vi "Fetch Waveform.vi"(0 "CS++Scope":refnum<class "CS++Scope.lvclass">, 1 "channel name (\"CHANNEL1\")":string="CHANNEL1", 2 "waveform size (0)":i32=1000, 5 "error in (no error)":errorcluster) -> (14 "CS++Scope out":refnum<class "CS++Scope.lvclass">, 15 "actual points":i32, 16 "initial x":dbl[unit] format="%^.2e", 17 "x increment":dbl[unit] format="%^.2e", 18 "WaveformArray":waveform(dbl), 19 "error out":errorcluster)   [LabVIEW 2014, in "CS++Scope.lvlib" / "CS++Scope.lvclass"]
doc: "This VI returns the waveform the oscilloscope acquires for the channel you specify. The waveform is from an acquisition that you initiate prior to calling this VI.\n\nThe VI also publishes a variable called MeasurementDone once all channels were updated since the last Init. Nevertheless one should still compare the time stamps of the acquired waveforms.\n\nYou use the IviScope Initiate Acquisition VI to start an acquisition on the channels that you enable with the IviScope Configure Channel VI. The oscilloscope acquires waveforms for the enabled channels concurrently. You use the IviScope Acquisition Status VI to determine when the acquisition is complete. You must call this VI separately for each enabled channel to obtain the waveforms.\n\nYou can call the IviScope Read Waveform VI instead of the IviScope Initiate Acquisition VI. The IviScope Read Waveform VI starts an acquisition on all enabled channels, waits for the acquisition to complete, and returns the waveform for the channel you specify. You call this VI to obtain the waveforms for each of the remaining channels.\n\nNotes:\n\n(1) After this VI executes, each element in the Waveform Array parameter is either a voltage or a value indicating that the oscilloscope could not sample a voltage.\n\n(2) You configure the interpolation method the oscilloscope uses with the IviScope Configure Interpolation [I] VI. If you disable interpolation, the oscilloscope does not interpolate points in the waveform. If the oscilloscope cannot sample a value for a point in the waveform, the driver sets the corresponding element in the Waveform Array to an IEEE defined NaN (Not a Number) value and the VI returns IVISCOPE_WARN_INVALID_WFM_ELEMENT (0x3FFA2001). \n\n(3) You can test a waveform value for an invalid value condition by calling the IviScope Is Invalid Waveform Element VI.\n\n(4) This VI does not check the instrument status. Typically, you call this VI only in a sequence of calls to other low-level driver VIs. The sequence performs one operation. You use the low-level VIs to optimize one or more aspects of interaction with the instrument. If you want to check the instrument status, call the IviScope Error-Query VI at the conclusion of the sequence.\n\n(5) The class driver returns a simulated waveform when this\nVI is called and the IviScope>>Inherent IVI Settings>>User Options>>Simulate property is set to TRUE and the IviScope>>Inherent IVI Settings>>User Options>>Use Specific Simulation property is set to FALSE. For information on how to configure a simulated waveform, refer to the online help manual."
uses:
  CS++Scope.lvclass
  CS++Scope.lvclass/CS++Scope.ctl
  CSPP_Core/Classes/CS++ProcessVariables/ProcessVariable/PV.lvclass
  PV-Enum.ctl
  CSPP_Core/Classes/CS++ProcessVariables/ProcessVariable/PV.lvclass/PV.ctl
  CSPP_Core/Classes/CS++ProcessVariables/ProcessVariable/Write Data.vi
  CSPP_Core/Classes/CS++ProcessVariables/ProcessVariable/Write Timestamp.vi
  CSPP_Core/Classes/CS++ProcessVariables/ProcessVariable/Write Quality.vi
  CSPP_Core/Classes/CS++ProcessVariables/ProcessVariable/Write status.vi
  CSPP_Core/Classes/CS++ProcessVariables/PVConnection/PVConnection.lvclass
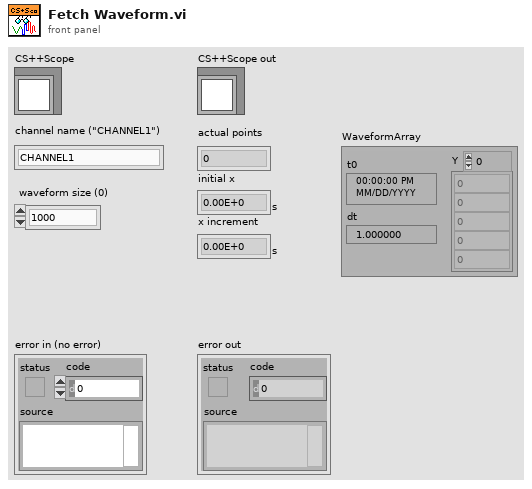
[diagram p1: front panel]
types:
  T1 = typedef "CS++Scope.lvlib/CS++Scope.lvclass/PV-Enum.ctl" = enum16{"ActualSampleRate", "TimePerRecord", "AcquisitionStartTime", "TriggerLevel", "GlitchWidth", "LowReference", "MidReference", "HighReference", "RuntLowThreshold", "RuntHighThreshold", "TriggerHoldoff", "WidthLowThreshold", "WidthHighThreshold", "AcquisitionStatus", "ActualRecordLength", "ActualSampleMode", "ACLineTriggerSlope", "MinRecordLength", "AcquisitionType", "TriggerSlope", "GlitchCondition", "GlitchPolarity", "InterpolationMethod", "NumberOfAverages", "NumberOfEnvelopes", "TriggerType", "TriggerCoupling", "TriggerModifier", "TVLineNumber", "TVEvent", "TVTriggerPolarity", "TVSignalFormat", "WidthCondition", "WidthPolarity", "MeasurementDone", "ContinousAcquisition", "TriggerSource", "Waveform", "ActualTimeIncrement"}
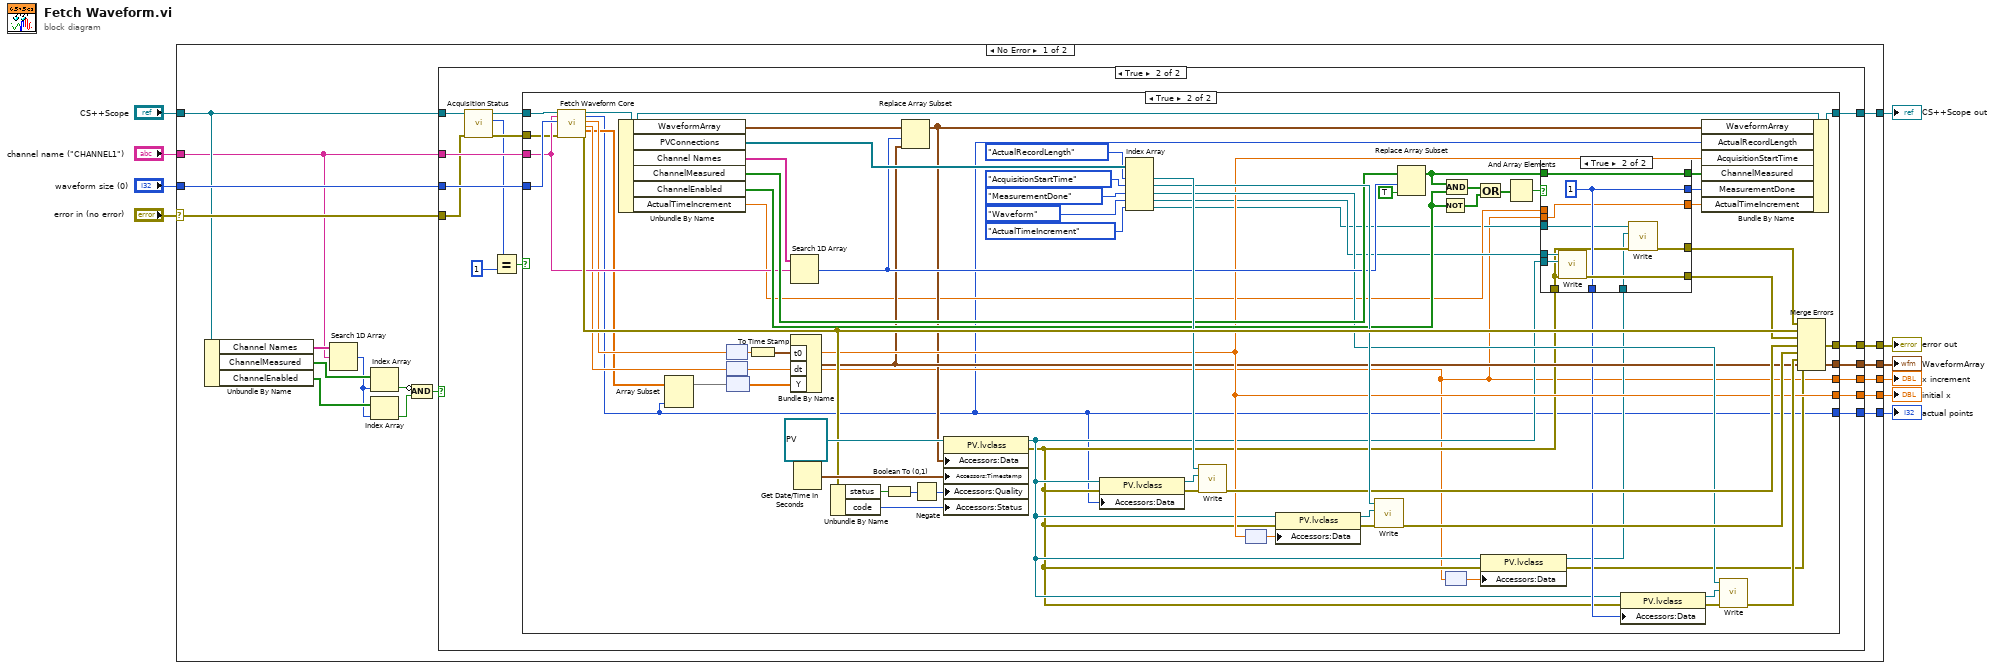
[diagram p0: block diagram]
diagram:
  n1 = case shown="No Error" "error in (no error)" {
    selector: "error in (no error)" -> [w27 w130]
    tunnel: [w26 w130] -> w9
    tunnel: [w22 w129] -> w6
    tunnel: "CS++Scope" -> [w19 w129]
    tunnel: "channel name (\"CHANNEL1\")" -> [w17 _]
    tunnel: "waveform size (0)" -> [w23 _]
    tunnel: [w21 _] -> w1
    tunnel: [w25 _] -> w4
    tunnel: [w20 _] -> w3
    tunnel: [w24 _] -> w2
    frame No Error {
      n2 = Unbundle By Name(w19) -> ("Channel Names"=w18:string[], "ChannelMeasured"=w16:bool[], "ChannelEnabled"=w15:bool[])
      n3 = Search 1D Array(1D array=w18, element=w17) -> (index of element=w14:i32)  [unwired: 1 in]
      n4 = Index Array(array=w16, index=w14) -> (element=w13:bool)
      n5 = Index Array(array=w15, index=w14) -> (element=w12:bool)
      n6 = Compound Arithmetic op=AND(invert w13, w12) -> (w11:bool)
      n7 = case shown="True" w11 {
        tunnel: w27 -> [w28 w34]
        tunnel: [w28 w44] -> w26
        tunnel: [_ w43] -> w25
        tunnel: [_ w42] -> w24
        tunnel: w23 -> [_ w41]
        tunnel: [w29 w40] -> w22
        tunnel: [_ w39] -> w21
        tunnel: [_ w38] -> w20
        tunnel: w19 -> [w29 w36]
        tunnel: w17 -> [_ w37]
        frame False {
        }
        frame True {
          n8 = call "Acquisition Status.vi"("error in (no error)"=w34, "CS++Scope"=w36) -> ("error out"=w33:errorcluster, "acquisition status"=w32:i32, "CS++Scope out"=w35:refnum<class "CS++Scope.lvclass">)  [unwired: 7 in]
          n9 = Equal?(x=w32, y=1) -> (x = y?=w30:bool)
          n10 = case shown="True" w30 {
            tunnel: [w46 w96] -> w44
            tunnel: [_ w47] -> w43
            tunnel: [_ w50] -> w42
            tunnel: w41 -> [_ w95]
            tunnel: [w45 w85] -> w40
            tunnel: [_ w68] -> w39
            tunnel: [_ w71] -> w38
            tunnel: w37 -> [_ w75]
            tunnel: w35 -> [w45 w74]
            tunnel: w33 -> [w46 w73]
            frame False {
            }
            frame True {
              n11 = call-dynamic "Fetch Waveform Core.vi"("CS++Scope"=w74, "channel name (\"CHANNEL1\")"=w75, "waveform size (0)"=w95, "error in (no error)"=w73) -> ("CS++Scope out"=w86:refnum<class "CS++Scope.lvclass">, "actual points"=w47:i32, "initial x"=w71:dbl[unit], "x increment"=w50:dbl[unit], "waveform array"=w49:dbl[unit][], "error out"=w107:errorcluster)  [unwired: 10 in]
              n12 = Unbundle By Name(w86) -> ("WaveformArray"=w114:waveform(dbl)[], "PVConnections"=w104:refnum<class "PVConnection.lvclass">[], "Channel Names"=w115:string[], "ChannelMeasured"=w94:bool[], "ChannelEnabled"=w91:bool[], "ActualTimeIncrement"=w60:dbl[unit])
              n13 = Array Subset(array=w49, length=w47) -> (w48:dbl[unit][])  [unwired: 1 in]
              n14 = node(w71) -> (w70:dbl)
              n15 = node(w50) -> (w59:dbl)
              n16 = node(w48) -> (w69:dbl[])
              n17 = To Time Stamp(1:w70) -> (0:w72:timestamp)
              n18 = Search 1D Array(1D array=w115, element=w75) -> (index of element=w93:i32)  [unwired: 1 in]
              n19 = Bundle By Name("t0"=w72, "dt"=w59, "Y"=w69) -> (w68:waveform(dbl))  [unwired: 1 in]
              n20 = Get Date/Time In Seconds() -> (seconds since 1Jan1904=w108:timestamp)
              n21 = Unbundle By Name(w107) -> ("status"=w111:bool, "code"=w112:i32)
              n22 = Boolean To (0,1)(Boolean=w111) -> (0, 1=w110:i16)
              n23 = Replace Array Subset(array=w114, new element=w68, index=w93) -> (w67:waveform(dbl)[])
              n24 = Negate(x=w110) -> (-x=w109:i16)
              n25 = property class="PV.lvclass"(reference=refnum<class "PV.lvclass"> refnum ("CS++ProcessVariables.lvlib:PV.lvclass"), "Accessors:Data"=w67, "Accessors:Timestamp"=w108, "Accessors:Quality"=w109, "Accessors:Status"=w112) -> (reference out=w55:refnum<class "PV.lvclass">, error out=w54:errorcluster)  [unwired: 1 in]
              n26 = property class="PV.lvclass"(reference=w55, error in=w54, "Accessors:Data"=w47) -> (reference out=w105:refnum<class "PV.lvclass">, error out=w106:errorcluster)
              n27 = Index Array(array=w104, index #1=PV-Enum."ActualRecordLength" ("PV-Enum"), index #2=PV-Enum."AcquisitionStartTime" ("PV-Enum"), index #3=PV-Enum."MeasurementDone" ("PV-Enum"), index #4=PV-Enum."Waveform" ("PV-Enum"), index #5=PV-Enum."ActualTimeIncrement" ("PV-Enum")) -> (element #1=w102:refnum<class "PVConnection.lvclass">, element #2=w99:refnum<class "PVConnection.lvclass">, element #3=w77:refnum<class "PVConnection.lvclass">, element #4=w63:refnum<class "PVConnection.lvclass">, element #5=w57:refnum<class "PVConnection.lvclass">)
              n28 = call-dynamic "Write.vi"("error in (no error)"=w106, "PV"=w105, "PVConnection in"=w102) -> ("error out"=w98:errorcluster)  [unwired: 7 in, 1 out]
              n29 = node(w71) -> (w76:dbl)
              n30 = property class="PV.lvclass"(reference=w55, error in=w54, "Accessors:Data"=w76) -> (reference out=w100:refnum<class "PV.lvclass">, error out=w101:errorcluster)
              n31 = call-dynamic "Write.vi"("error in (no error)"=w101, "PV"=w100, "PVConnection in"=w99) -> ("error out"=w97:errorcluster)  [unwired: 7 in, 1 out]
              n32 = Replace Array Subset(array=w94, new element=TRUE ("new element/subarray"), index=w93) -> (w83:bool[])
              n33 = Not(x=w91) -> (.not. x?=w89:bool[])
              n34 = node(w50) -> (w51:dbl)
              n35 = Compound Arithmetic op=AND(w83, w91) -> (w90:bool[])
              n36 = Or(x=w90, y=w89) -> (x .or. y?=w88:bool[])
              n37 = property class="PV.lvclass"(reference=w55, error in=w54, "Accessors:Data"=w51) -> (reference out=w52:refnum<class "PV.lvclass">, error out=w53:errorcluster)
              n38 = And Array Elements(Boolean array=w88) -> (logical AND=w87:bool)
              n39 = case shown="True" w87 {
                tunnel: [w118 w128] -> w84
                tunnel: w83 -> [w118 w128]
                tunnel: [_ w124] -> w79
                tunnel: w63 -> [_ w127]
                tunnel: [w117 w126] -> w66
                tunnel: w54 -> [w117 w120]
                tunnel: w55 -> [_ w125]
                tunnel: [_ w124] -> w61
                tunnel: w60 -> [w116 _]
                tunnel: w50 -> [_ w123]
                tunnel: [w116 w123] -> w58
                tunnel: w57 -> [_ w122]
                tunnel: [_ w121] -> w56
                tunnel: w52 -> [_ w119]
                frame False {
                }
                frame True {
                  w124 = 1 ("MeasurementDone")
                  n40 = call-dynamic "Write.vi"("error in (no error)"=w120, "PV"=w125, "PVConnection in"=w127) -> ("error out"=w126:errorcluster)  [unwired: 7 in, 1 out]
                  n41 = call-dynamic "Write.vi"("error in (no error)"=w120, "PV"=w119, "PVConnection in"=w122) -> ("error out"=w121:errorcluster)  [unwired: 7 in, 1 out]
                }
              }
              n42 = property class="PV.lvclass"(reference=w55, error in=w54, "Accessors:Data"=w61) -> (reference out=w80:refnum<class "PV.lvclass">, error out=w81:errorcluster)
              n43 = Bundle By Name(cluster=w86, "WaveformArray"=w67, "ActualRecordLength"=w47, "AcquisitionStartTime"=w71, "ChannelMeasured"=w84, "MeasurementDone"=w79, "ActualTimeIncrement"=w58) -> (w85:refnum<class "CS++Scope.lvclass">)
              n44 = call-dynamic "Write.vi"("error in (no error)"=w81, "PV"=w80, "PVConnection in"=w77) -> ("error out"=w78:errorcluster)  [unwired: 7 in, 1 out]
              n45 = Merge Errors(w56, w107, w66, w98, w97, w78, w53) -> (w96:errorcluster)
            }
          }
        }
      }
    }
    frame Error {
    }
  }
  "error out" <- w9
  "actual points" <- w4
  "initial x" <- w3
  "x increment" <- w2
  "CS++Scope out" <- w6
  "WaveformArray" <- w1
